vi "Plot 366.vi"() -> ()   [LabVIEW 2017]
uses:
  <vilib>/Utility/file.llb/Read Delimited Spreadsheet (DBL).vi
  <vilib>/Analysis/NI_AALBase.lvlib
  <vilib>/gmath/NI_Gmath.lvlib
panel:
  out "Ready?":bool=TRUE
  in  "Auto x axis T":bool
  in  "Tab Control 2":enum32{"Contour", "Curve"}(tab)
  out "Intensity Graph":dbl[][](graph)
  out "XY Graph":cluster{"Y":dbl[], "Y":dbl[]}[](graph)=[{"Y"=[0.0, 0.05, 0.1, 0.15, 0.2, 0.25, 0.3, 0.35, 0.4, 0.45, 0.5, 0.55, 0.6, 0.65, 0.7, 0.75, 0.8, 0.85, 0.9, 0.95, 1.0, 1.05, 1.1, 1.15, 1.2, 1.25, 1.3, 1.35, 1.4, 1.45, 1.5, 1.55, 1.6, 1.55, 1.5, 1.45, 1.4, 1.35, 1.3, 1.25, 1.2, 1.15, 1.1, 1.05, 1.0, 0.95, 0.9, 0.85, 0.8, 0.75, 0.7, 0.65, 0.6, 0.55, 0.5, 0.45, 0.4, 0.35, 0.3, 0.25, 0.2, 0.15, 0.1, 0.05, 0.0, -0.05, -0.1, -0.15, -0.2, -0.25, -0.3, -0.35, -0.4, -0.45, -0.5, -0.55, -0.6, -0.65, -0.7, -0.75, -0.8, -0.85, -0.9, -0.95, -1.0, -1.05, -1.1, -1.15, -1.2, -1.25, -1.3, -1.35, -1.4, -1.45, -1.5, -1.55, -1.6, -1.55, -1.5, -1.45, -1.4, -1.35, -1.3, -1.25, -1.2, -1.15, -1.1, -1.05, -1.0, -0.95, -0.9, -0.85, -0.8, -0.75, -0.7, -0.65, -0.6, -0.55, -0.5, -0.45, -0.4, -0.35, -0.3, -0.25, -0.2, -0.15, -0.1, -0.05], "Y"=[-inf, -inf, -inf, -inf, -inf, -inf, -inf, 3.5817700050999997, -inf, -inf, -inf, -inf, -inf, -inf, -inf, -inf, -inf, -inf, -inf, -inf, -inf, -inf, -inf, -inf, -inf, -inf, -inf, -inf, -inf, -inf, -inf, -inf, -inf, -inf, -inf, -inf, -inf, -inf, -inf, -inf, -inf, -inf, -inf, -inf, -inf, -inf, -inf, -inf, -inf, -inf, -inf, -inf, -inf, -inf, -inf, -inf, -inf, -inf, -inf, -inf, -inf, -inf, -inf, -inf, -inf, -inf, -inf, -inf, -inf, -inf, -inf, -inf, -inf, -inf, -inf, -inf, -inf, -inf, -inf, -inf, -inf, -inf, -inf, -inf, -inf, -inf, -inf, -inf, -inf, -inf, -inf, -inf, 0.5863699898000001, -inf, -inf, -inf, -inf, -inf, -inf, -inf, 0.6016699898, -inf, -inf, -inf, -inf, -inf, -inf, -inf, -inf, -inf, -inf, -inf, -inf, -inf, -inf, -inf, -inf, -inf, -inf, -inf, -inf, -inf, -inf, -inf, -inf, -inf, -inf, -inf]}]
  in  "Voltage treshold":dbl=1.2e-05 format="%_3g"
  in  "Ignore points":i32=250
  in  "Tab Control":enum32{"Y cut ", "Y curve", "X cut"}(tab)=enum."Y curve"
  out "Y Cut":cluster{dbl[], "Intensity Graph":dbl[]}(graph)
  in  "intervals":i32=100
  out "Y Histogram":T1(graph)={"X Values"=[3.561031115, 3.562637345, 3.5642435750000003, 3.5658498050000005, 3.5674560350000006, 3.569062265000001, 3.570668495000001, 3.572274725000001, 3.5738809550000012, 3.5754871850000014, 3.5770934150000016, 3.5786996450000017, 3.580305875000002, 3.581912105000002, 3.583518335000002, 3.5851245650000023, 3.5867307950000025, 3.5883370250000026, 3.5899432550000028, 3.591549485000003, 3.593155715000003, 3.5947619450000032, 3.5963681750000034, 3.5979744050000035, 3.5995806350000037, 3.601186865000004, 3.602793095000004, 3.604399325000004, 3.6060055550000043, 3.6076117850000045, 3.6092180150000046, 3.6108242450000048, 3.612430475000005, 3.614036705000005, 3.615642935000005, 3.6172491650000054, 3.6188553950000055, 3.6204616250000057, 3.622067855000006, 3.623674085000006, 3.625280315000006, 3.6268865450000063, 3.6284927750000064, 3.6300990050000066, 3.6317052350000067, 3.633311465000007, 3.634917695000007, 3.636523925000007, 3.6381301550000074, 3.6397363850000075, 3.6413426150000077, 3.642948845000008, 3.644555075000008, 3.646161305000008, 3.6477675350000083, 3.6493737650000084, 3.6509799950000086, 3.6525862250000087, 3.654192455000009, 3.655798685000009, 3.657404915000009, 3.6590111450000093, 3.6606173750000095, 3.6622236050000097, 3.66382983500001, 3.66543606500001, 3.66704229500001, 3.6686485250000103, 3.6702547550000104, 3.6718609850000106, 3.6734672150000107, 3.675073445000011, 3.676679675000011, 3.678285905000011, 3.6798921350000113, 3.6814983650000115, 3.6831045950000116, 3.684710825000012, 3.686317055000012, 3.687923285000012, 3.6895295150000122, 3.6911357450000124, 3.6927419750000126, 3.6943482050000127, 3.695954435000013, 3.697560665000013, 3.699166895000013, 3.7007731250000133, 3.7023793550000135, 3.7039855850000136, 3.7055918150000138, 3.707198045000014, 3.708804275000014, 3.7104105050000142, 3.7120167350000144, 3.7136229650000145, 3.7152291950000147, 3.716835425000015, 3.718441655000015, 3.720047885000015], "Histogram: h(x)"=[1, 0, 1, 0, 0, 0, 1, 2, 0, 1, 0, 0, 1, 0, 0, 0, 4, 1, 2, 3, 0, 3, 2, 1, 2, 5, 4, 6, 4, 9, 5, 14, 9, 11, 9, 12, 10, 9, 21, 15, 22, 22, 26, 27, 35, 33, 39, 44, 46, 39, 55, 71, 80, 86, 91, 108, 113, 124, 104, 148, 162, 170, 189, 195, 222, 265, 248, 282, 257, 305, 311, 307, 293, 347, 370, 337, 349, 396, 361, 353, 349, 336, 303, 309, 292, 254, 217, 183, 154, 133, 89, 71, 47, 27, 14, 10, 7, 3, 1, 1]}
  out "X Cut":cluster{dbl[], "Intensity Graph":dbl[]}(graph)={[0.0, 0.05, 0.1, 0.15000000000000002, 0.2, 0.25, 0.30000000000000004, 0.35000000000000003, 0.4, 0.45, 0.5, 0.55, 0.6000000000000001, 0.65, 0.7000000000000001, 0.75, 0.8, 0.8500000000000001, 0.9, 0.9500000000000001, 1.0, 1.05, 1.1, 1.1500000000000001, 1.2000000000000002, 1.25, 1.3, 1.35, 1.4000000000000001, 1.4500000000000002, 1.5, 1.55, 1.6, 1.6500000000000001, 1.7000000000000002, 1.75, 1.8, 1.85, 1.9000000000000001, 1.9500000000000002, 2.0, 2.0500000000000003, 2.1, 2.15, 2.2, 2.25, 2.3000000000000003, 2.35, 2.4000000000000004, 2.45, 2.5, 2.5500000000000003, 2.6, 2.6500000000000004, 2.7, 2.75, 2.8000000000000003, 2.85, 2.9000000000000004, 2.95, 3.0, 3.0500000000000003, 3.1, 3.1500000000000004, 3.2, 3.25, 3.3000000000000003, 3.35, 3.4000000000000004, 3.45, 3.5, 3.5500000000000003, 3.6, 3.6500000000000004, 3.7, 3.75, 3.8000000000000003, 3.85, 3.9000000000000004, 3.95, 4.0, 4.05, 4.1000000000000005, 4.15, 4.2, 4.25, 4.3, 4.3500000000000005, 4.4, 4.45, 4.5, 4.55, 4.6000000000000005, 4.65, 4.7, 4.75, 4.800000000000001, 4.8500000000000005, 4.9, 4.95, 5.0, 5.050000000000001, 5.1000000000000005, 5.15, 5.2, 5.25, 5.300000000000001, 5.3500000000000005, 5.4, 5.45, 5.5, 5.550000000000001, 5.6000000000000005, 5.65, 5.7, 5.75, 5.800000000000001, 5.8500000000000005, 5.9, 5.95, 6.0, 6.050000000000001, 6.1000000000000005, 6.15, 6.2, 6.25, 6.300000000000001, 6.3500000000000005], "Intensity Graph"=[0.0, 0.0, 0.0, 0.0, 0.0, 0.0, 0.0, 0.0, 0.0, 0.0, 0.0, 0.0, 0.0, 0.0, 0.0, 0.0, 0.0, 0.0, 0.0, 0.0, 0.0, 0.0, 0.0, 0.0, 0.0, 0.0, 0.0, 0.0, 0.0, 0.0, 0.0, 0.0, 0.0, 0.0, 0.0, 0.0, 0.0, 0.0, 0.0, 0.0, 2.0, 0.0, 0.0, 0.0, 0.0, 0.0, 0.0, 0.0, 0.0, 0.0, 0.0, 0.0, 0.0, 0.0, 0.0, 0.0, 0.0, 0.0, 0.0, 0.0, 0.0, 0.0, 0.0, 0.0, 0.0, 0.0, 0.0, 0.0, 0.0, 0.0, 0.0, 0.0, 0.0, 0.0, 0.0, 0.0, 0.0, 0.0, 0.0, 2.0, 0.0, 0.0, 0.0, 0.0, 0.0, 0.0, 0.0, 0.0, 0.0, 0.0, 0.0, 0.0, 0.0, 0.0, 0.0, 0.0, 0.0, 0.0, 0.0, 0.0, 0.0, 0.0, 0.0, 0.0, 0.0, 0.0, 0.0, 0.0, 0.0, 0.0, 61.0, 0.0, 0.0, 0.0, 0.0, 0.0, 0.0, 0.0, 0.0, 0.0, 0.0, 0.0, 0.0, 0.0, 0.0, 0.0, 0.0, 0.0]}
  in  "Normal T or Distribution F":bool
  in  "book number":i32=366
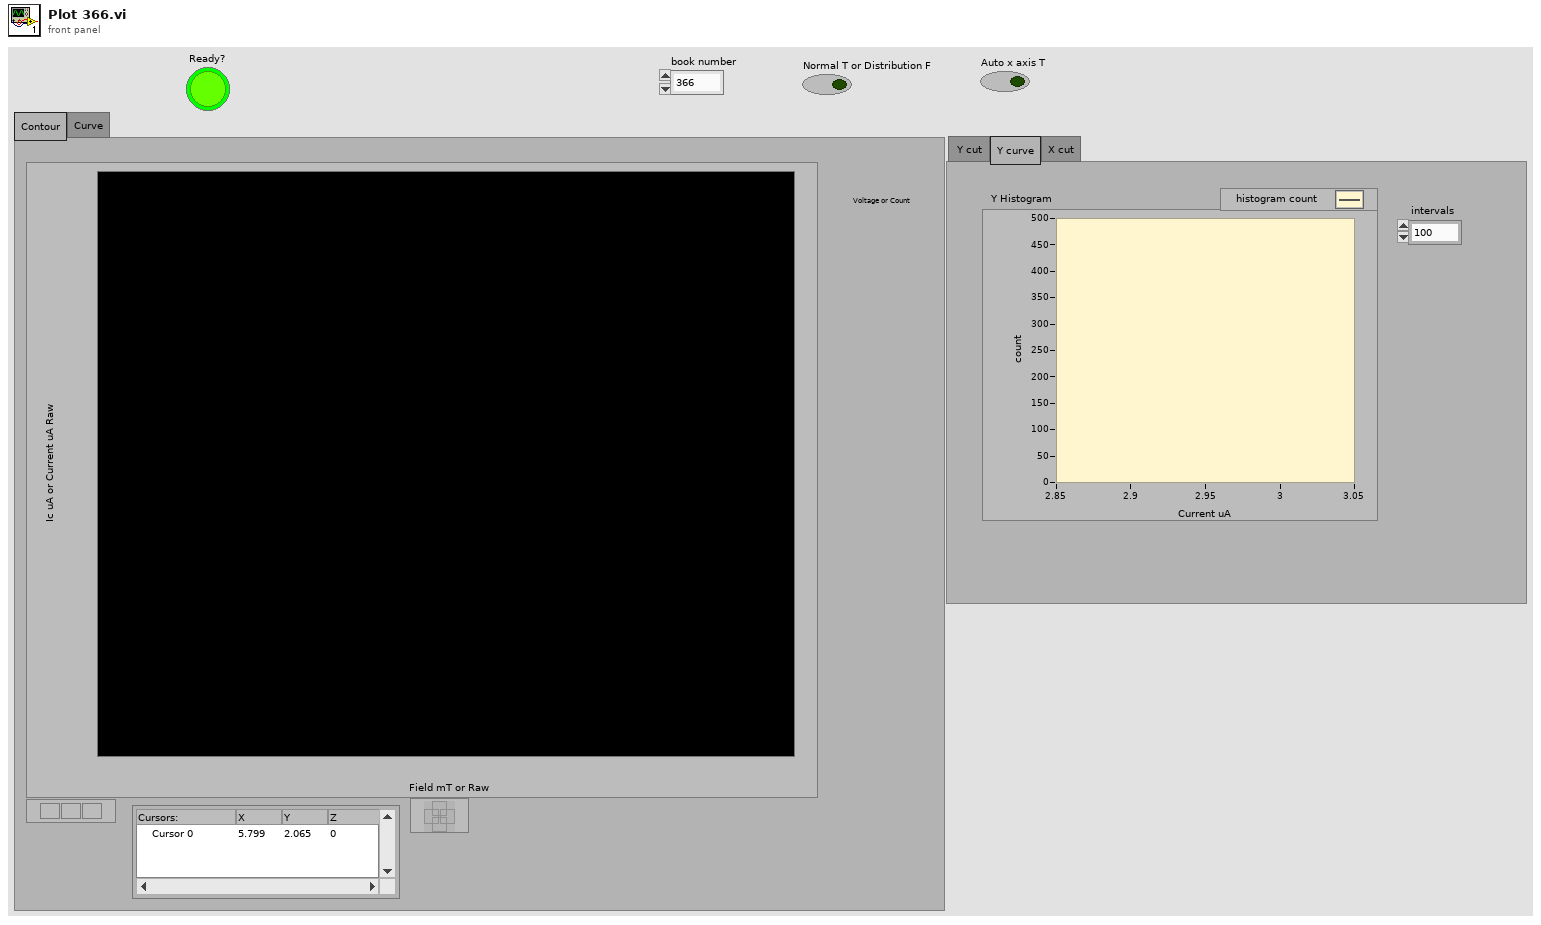
[diagram p1: front panel]
types:
  T1 = cluster{"X Values":dbl[], "Histogram: h(x)":i32[]}
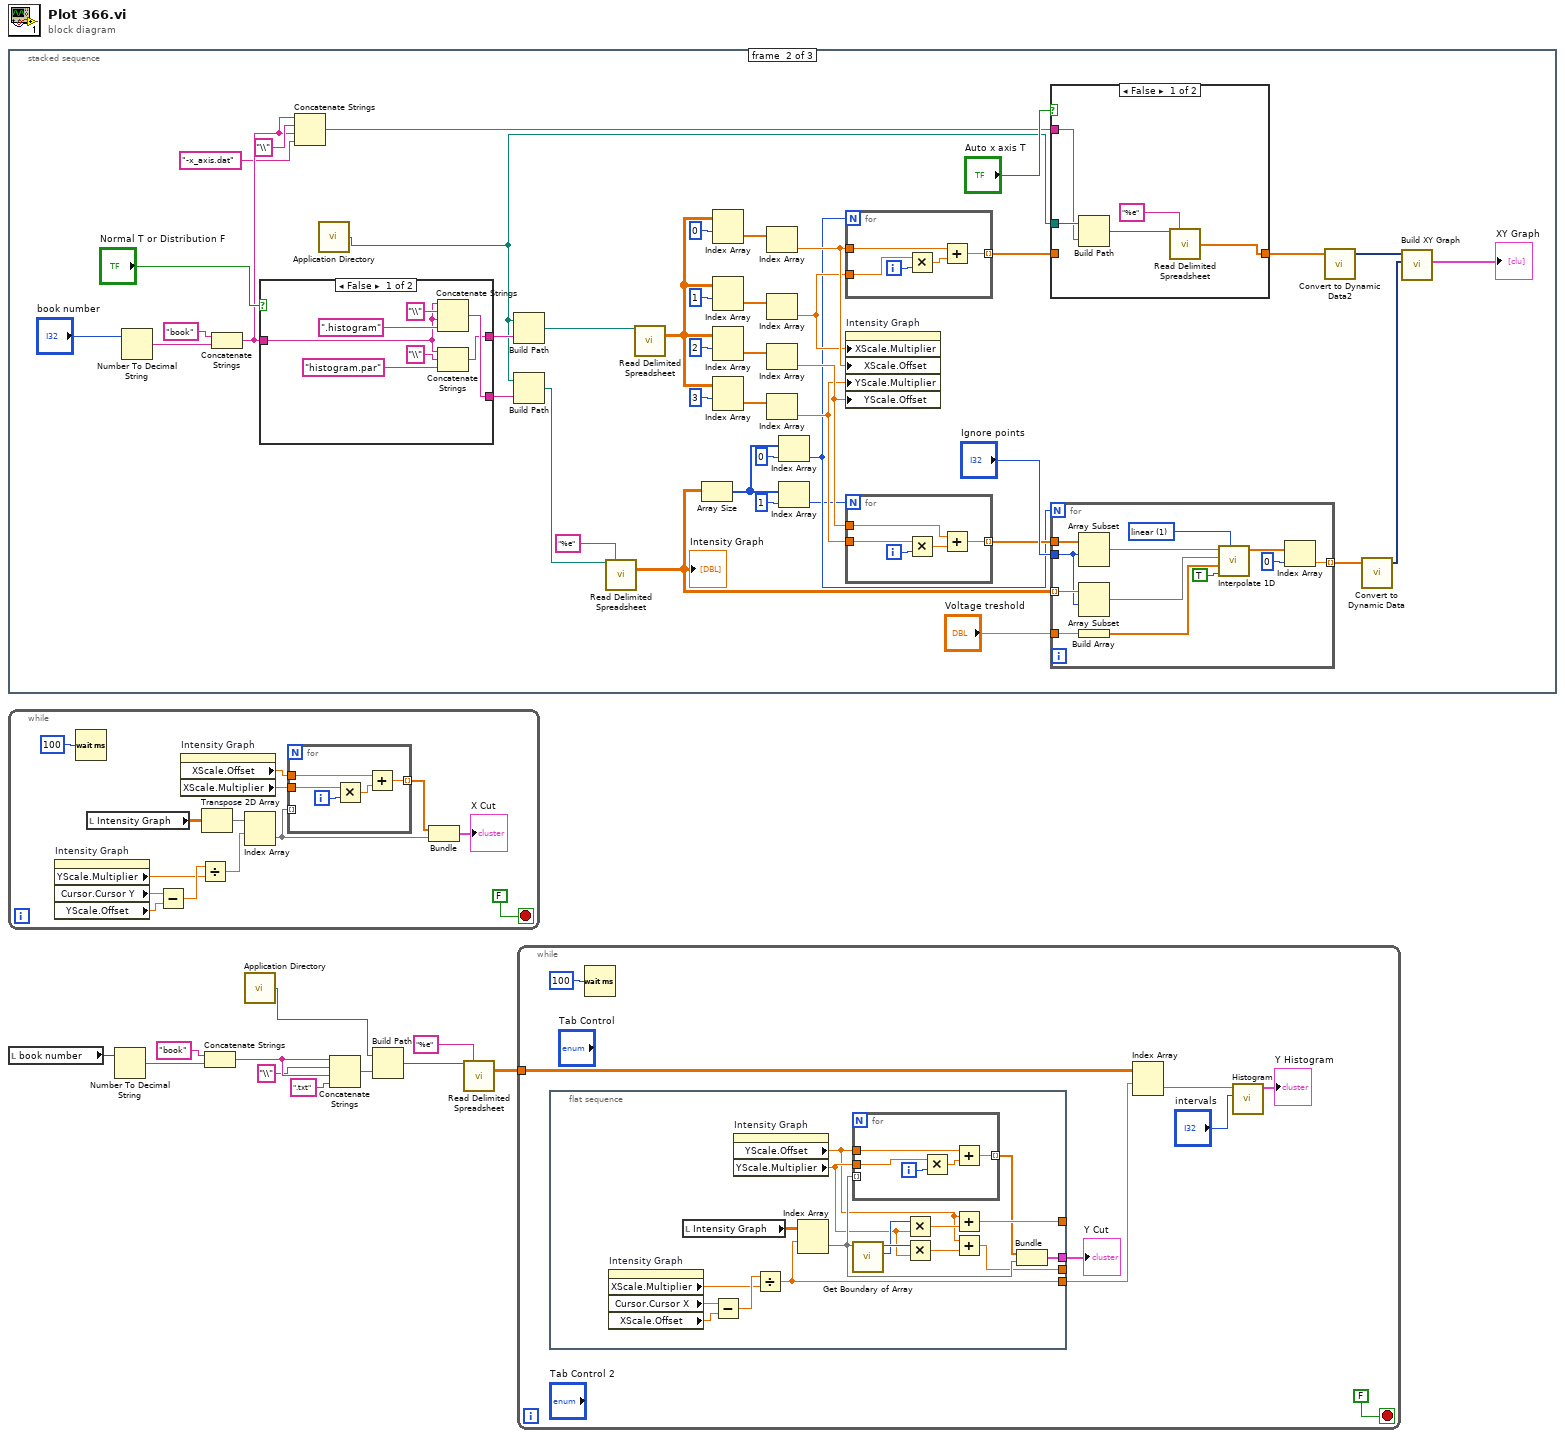
[diagram p0: block diagram]
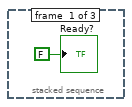
[diagram p2: hidden frame]
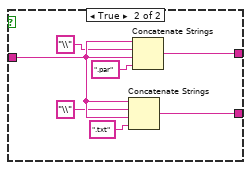
[diagram p4: hidden frame]
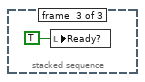
[diagram p5: hidden frame]
diagram:
  n1 = stacked-sequence {
    frame #0 {
      "Ready?" <- FALSE ("Ready?")
    }
    frame #1 {
      n2 = Number To Decimal String(number="book number") -> (decimal integer string=w51:string)  [unwired: 1 in]
      n3 = Concatenate Strings("book" ("string"), w51) -> (w20:string)
      n4 = case shown="False" "Normal T or Distribution F" {
        tunnel: [w86 w97] -> w53
        tunnel: w20 -> [w85 w95]
        tunnel: [w87 w93] -> w52
        frame False {
          n5 = Concatenate Strings(w85, "\\" ("string"), w85, ".histogram" ("string")) -> (w87:string)
          n6 = Concatenate Strings(w85, "\\" ("string"), "histogram.par" ("string")) -> (w86:string)
        }
        frame True {
          n7 = Concatenate Strings(w95, "\\" ("string"), w95, ".txt" ("string")) -> (w93:string)
          n8 = Concatenate Strings(w95, "\\" ("string"), w95, ".par" ("string")) -> (w97:string)
        }
      }
      n9 = Concatenate Strings(w20, "\\" ("string"), w20, "-x_axis.dat" ("string")) -> (w18:string)
      n10 = call <vilib>:"Application Directory.vi"() -> ("Application Directory"=w13:path)
      n11 = Build Path(base path=w13, name or relative path=w53) -> (appended path=w54:path)
      n12 = Build Path(base path=w13, name or relative path=w52) -> (appended path=w55:path)
      n13 = call-poly <vilib>:"Read Delimited Spreadsheet.vi"("file path (dialog if empty)"=w55, "format (%.3f)"="%e") -> ("all rows"=w37:dbl[][])  [unwired: 8 in, 5 out]
      "Intensity Graph" <- w37
      n14 = call-poly <vilib>:"Read Delimited Spreadsheet.vi"("file path (dialog if empty)"=w54) -> ("all rows"=w47:dbl[][])  [unwired: 9 in, 5 out]
      n15 = Array Size(array=w37) -> (size(s)=w17:i32[])
      n16 = Index Array(array=w47, index (row)=0) -> (element=w44:dbl[])  [unwired: 1 in]
      n17 = Index Array(array=w47, index (row)=1) -> (element=w43:dbl[])  [unwired: 1 in]
      n18 = Index Array(array=w47, index (row)=2) -> (element=w42:dbl[])  [unwired: 1 in]
      n19 = Index Array(array=w47, index (row)=3) -> (element=w41:dbl[])  [unwired: 1 in]
      n20 = Index Array(array=w44) -> (element=w34:dbl)  [unwired: 1 in]
      n21 = Index Array(array=w43) -> (element=w33:dbl)  [unwired: 1 in]
      n22 = Index Array(array=w42) -> (element=w36:dbl)  [unwired: 1 in]
      n23 = Index Array(array=w41) -> (element=w35:dbl)  [unwired: 1 in]
      n24 = Index Array(array=w17, index=0) -> (element=w15:i32)
      n25 = Index Array(array=w17, index=1) -> (element=w14:i32)
      n26 = for {
        N: w15 -> [_]
        tunnel: w34 -> [w66]
        tunnel: w33 -> [w64]
        tunnel: [w62] -> w23 mode=indexing
        i -> [w65]
        n27 = Multiply(x=w64, y=w65) -> (x*y=w63:dbl)
        n28 = Add(x=w66, y=w63) -> (x+y=w62:dbl)
      }
      n29 = property on="Intensity Graph" class="IntGraph (strict)"("XScale.Multiplier"=w33, "XScale.Offset"=w34, "YScale.Multiplier"=w35, "YScale.Offset"=w36) -> ()  [unwired: 2 in, 2 out]
      n30 = for {
        N: w14 -> [_]
        tunnel: w36 -> [w71]
        tunnel: w35 -> [w69]
        tunnel: [w67] -> w25 mode=indexing
        i -> [w70]
        n31 = Multiply(x=w69, y=w70) -> (x*y=w68:dbl)
        n32 = Add(x=w71, y=w68) -> (x+y=w67:dbl)
      }
      n33 = case shown="False" "Auto x axis T" {
        tunnel: w23 -> [_ w61]
        tunnel: [w56 w61] -> w22
        tunnel: w13 -> [w60 _]
        tunnel: w18 -> [w59 _]
        frame False {
          n34 = Build Path(base path=w60, name or relative path=w59) -> (appended path=w58:path)
          n35 = call-poly <vilib>:"Read Delimited Spreadsheet.vi"("file path (dialog if empty)"=w58, "format (%.3f)"="%e") -> ("first row"=w56:dbl[])  [unwired: 8 in, 5 out]
        }
        frame True {
        }
      }
      n36 = for {
        N: w15 -> [_]
        tunnel: w37 -> [w76] mode=indexing
        tunnel: w25 -> [w77]
        tunnel: [w78] -> w31 mode=indexing
        tunnel: "Ignore points" -> [w72]
        tunnel: "Voltage treshold" -> [w73]
        w82 = 1 items=["nearest", "linear", "spline", "cubic Hermite", "Lagrange"] ("method")
        n37 = Array Subset(array=w77, index=w72) -> (w74:dbl[])  [unwired: 1 in]
        n38 = Array Subset(array=w76, index=w72) -> (w75:dbl[])  [unwired: 1 in]
        n39 = Build Array(w73) -> (w81:dbl[])
        n40 = call <vilib>:"Interpolate 1D.vi"("method"=w82, "X is monotonic"=TRUE, "xi"=w81, "X"=w75, "Y"=w74) -> ("yi"=w80:dbl[])  [unwired: 4 in, 2 out]
        n41 = Index Array(array=w80, index=0) -> (element=w78:dbl)
      }
      n42 = call "Convert to Dynamic Data2"("Array"=w22) -> ("Dynamic Data Type"=w29:dynamicdata)  [unwired: 3 in]
      n43 = call "Convert to Dynamic Data"("Array"=w31) -> ("Dynamic Data Type"=w30:dynamicdata)  [unwired: 3 in]
      n44 = call "Build XY Graph"("Y Input"=w30, "X Input"=w29) -> ("XY Graph"=→"XY Graph":cluster{"X":dbl[], "Y":dbl[]}[])  [unwired: 8 in, 1 out]
    }
    frame #2 {
      n45 = local write "Ready?"(TRUE ("Ready?")) -> ()
    }
  }
  n46 = while {
    stop <- FALSE stop-if-true
    n47 = property on="Intensity Graph" class="IntGraph (strict)"() -> ("YScale.Multiplier"=w107:dbl, "Cursor.Cursor Y"=w106:dbl, "YScale.Offset"=w105:dbl)  [unwired: 2 in, 2 out]
    n48 = Wait (ms)(milliseconds to wait=u32 100) -> ()  [unwired: 1 out]
    n49 = local read "Intensity Graph"() -> (w102:dbl[][])
    n50 = Subtract(x=w106, y=w105) -> (x-y=w112:dbl)
    n51 = property on="Intensity Graph" class="IntGraph (strict)"() -> ("XScale.Offset"=w108:dbl, "XScale.Multiplier"=w109:dbl)  [unwired: 2 in, 2 out]
    n52 = Divide(x=w112, y=w107) -> (x/y=w111:dbl)
    n53 = Transpose 2D Array(2D array=w102) -> (transposed array=w101:dbl[][])
    n54 = Index Array(array=w101, index (row)=w111) -> (element=w103:dbl[])  [unwired: 1 in]
    n55 = for {
      tunnel: w109 -> [w116]
      tunnel: w108 -> [w114]
      tunnel: [w113] -> w110 mode=indexing
      tunnel: w103 -> [_] mode=indexing
      i -> [w117]
      n56 = Multiply(x=w116, y=w117) -> (x*y=w115:dbl)
      n57 = Add(x=w114, y=w115) -> (x+y=w113:dbl)
    }
    n58 = Bundle(w110, w103) -> (→"X Cut":cluster{dbl[], dbl[]})  [unwired: 1 in]
  }
  n59 = local read "book number"() -> (w7:i32)
  n60 = Number To Decimal String(number=w7) -> (decimal integer string=w6:string)  [unwired: 1 in]
  n61 = Concatenate Strings("book" ("string"), w6) -> (w8:string)
  n62 = call <vilib>:"Application Directory.vi"() -> ("Application Directory"=w1:path)
  n63 = Concatenate Strings(w8, "\\" ("string"), w8, ".txt" ("string")) -> (w9:string)
  n64 = Build Path(base path=w1, name or relative path=w9) -> (appended path=w10:path)
  n65 = call-poly <vilib>:"Read Delimited Spreadsheet.vi"("file path (dialog if empty)"=w10, "format (%.3f)"="%e") -> ("all rows"=w11:dbl[][])  [unwired: 8 in, 5 out]
  n66 = while {
    tunnel: w11 -> [w121]
    stop <- FALSE stop-if-true
    n67 = flat-sequence {
      tunnel: [w137] -> w125
      tunnel: [w129] -> _
      tunnel: [w128] -> _
      tunnel: [w127] -> w122
      frame #0 {
        n68 = property on="Intensity Graph" class="IntGraph (strict)"() -> ("XScale.Multiplier"=w140:dbl, "Cursor.Cursor X"=w139:dbl, "XScale.Offset"=w138:dbl)  [unwired: 2 in, 2 out]
        n69 = local read "Intensity Graph"() -> (w141:dbl[][])
        n70 = Subtract(x=w139, y=w138) -> (x-y=w142:dbl)
        n71 = property on="Intensity Graph" class="IntGraph (strict)"() -> ("YScale.Offset"=w130:dbl, "YScale.Multiplier"=w131:dbl)  [unwired: 2 in, 2 out]
        n72 = Divide(x=w142, y=w140) -> (x/y=w127:dbl)
        n73 = Index Array(array=w141, index (row)=w127) -> (element=w136:dbl[])  [unwired: 1 in]
        n74 = for {
          tunnel: w131 -> [w146]
          tunnel: w130 -> [w144]
          tunnel: [w143] -> w126 mode=indexing
          tunnel: w136 -> [_] mode=indexing
          i -> [w147]
          n75 = Multiply(x=w146, y=w147) -> (x*y=w145:dbl)
          n76 = Add(x=w144, y=w145) -> (x+y=w143:dbl)
        }
        n77 = call "Get Boundary of Array.vi"("Array"=w136) -> ("Up"=w132:i32, "Down"=w135:i32)  [unwired: 9 in]
        n78 = Multiply(x=w132, y=w131) -> (x*y=w133:dbl)
        n79 = Multiply(x=w135, y=w131) -> (x*y=w134:dbl)
        n80 = Add(x=w130, y=w133) -> (x+y=w128:dbl)
        n81 = Add(x=w130, y=w134) -> (x+y=w129:dbl)
        n82 = Bundle(w126, "Intensity Graph"=w136) -> (w137:cluster{dbl[], "Intensity Graph":dbl[]})  [unwired: 1 in]
      }
    }
    n83 = Wait (ms)(milliseconds to wait=u32 100) -> ()  [unwired: 1 out]
    n84 = Index Array(array=w121, index (row)=w122) -> (element=w120:dbl[])  [unwired: 1 in]
    n85 = call <vilib>:"Histogram.vi"("intervals"="intervals", "X"=w120) -> ("Histogram Graph"=→"Y Histogram":T1)  [unwired: 6 in, 3 out]
    "Y Cut" <- w125
  }
